vi "UiCharts24h_b2g2.vi"() -> ()   [LabVIEW 2011]
uses:
  Output - Cluster b2g2.ctl
  Input - Cluster b2g2.ctl
  <vilib>/Platform/TimedLoop/XDataNode/timing_clust.ctl
  <vilib>/Platform/TimedLoop/XDataNode/nitl_modes.ctl
  <vilib>/Platform/TimedLoop/XDataNode/wakeup.ctl
  <vilib>/addons/database/Connection.llb/DB Tools Open Connec (String).vi
  <vilib>/addons/database/Connection.llb/Conn Execute.vi
  <vilib>/addons/database/Recordset.llb/Rec Fetch Recordset Data (R).vi
  <vilib>/addons/database/Recordset.llb/Rec Destroy - Connection.vi
  <vilib>/Platform/TimedLoop/XDataNode/XDataNode.xnode
  <vilib>/addons/database/_DB Variant To Data/Database Variant To Data.xnode
  <vilib>/addons/database/NI_Database_API.lvlib
  <vilib>/Platform/TimedLoop/XDataNode/XDNodeRunTimeDep.lvlib
panel:
  in  "Output Var":refnum<k21>="ni.var.psp://10.27.40.21/variables - b2g2/data - network b2g2"
  in  "Input Var":refnum<k21>="ni.var.psp://10.27.40.21/variables - b2g2/input - network b2g2"
  in  "Tab Control":T1(tab)
  out "protocol":string[][](table)
  out "pH-Wert":dbl(graph)
  out "Temperaturregelung":T2(graph)
  out "Füllstandsregelung":T3(graph)
  out "Druckregelung":T4(graph)
  out "error out":errorcluster
  in  "stop":bool
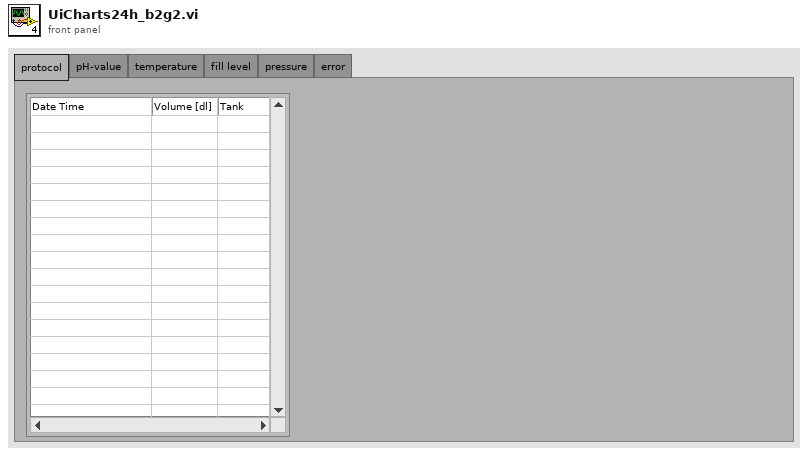
[diagram p1: front panel]
types:
  T1 = enum32{"protocol", "pH-value", "temperature", "fill level", "pressure", "error"}
  T2 = cluster{"Temp Soll [°C]":sgl, "TS-4 [°C]":dbl, dbl, dbl}
  T3 = cluster{"Füllstand Soll [l]":sgl, "FS-3 [l]":dbl, dbl}
  T4 = cluster{"Druck Soll [bar]":sgl, "DS-1 [bar]":dbl, dbl, dbl}
  T5 = typedef "Input - Cluster b2g2.ctl" = cluster{"V-13 [%]":u8, "V-15 [%]":u8, "Log-Target":bool, "P-4":bool, "P-4 Drehzahl [%]":u8, "Temperaturregelung":bool, "Überdruckregelung":bool, "Füllstandsregulierung":bool, "V-10":bool, "Log-Host":bool, "V-14":bool, "HS-1":bool, "Füllstand  P":sgl, "Füllstand I":sgl, "Füllstand D":sgl, "Füllstand Soll [l]":sgl, "Druck  P":sgl, "Druck I":sgl, "Druck D":sgl, "Druck Soll [bar]":sgl, "Temp Soll [°C]":sgl, "Dosierung":bool, "Dosiermenge [l]":sgl, "Dosiergeschw. [l/min]":sgl, "Tank":bool, "Hysterese [°C]":sgl, "MR Füllstandsüberwachung":bool, "Tank Füllstandsüberwachung":bool, "Log Target [ms]":u32, "Log Host [s]":u32, "Zirkulation EIN [min]":u8, "Zirkulation AUS [min]":u8, "Zirkulation":bool, "V-33":bool, "V-34":bool, "V-35":bool}
  T6 = typedef "Output - Cluster b2g2.ctl" = cluster{"DFS-1 [dl]":u64, "FS-3 [l]":dbl, "DFS-1 [l/min]":dbl, "DS-1 [bar]":dbl, "V-10 ZU":bool, "V-14 ZU":bool, "FS-1 [l]":dbl, "FS-2 [l]":dbl, "TS-4 [°C]":dbl, "HS-1":bool, "V-13 [%]":u8, "V-15 [%]":u8, "P-4 [%]":u8, "Dosierung":bool, "MR Max Füllstand":bool, "MR Min Füllstand":bool, "Dosiermenge [l]":sgl, "V-14 AUF":bool, "V-10 AUF":bool, "T-1 Max Füllstand":bool, "T-1 Min Füllstand":bool, "T-2 Max Füllstand":bool, "T-2 Min Füllstand":bool, "pHS-1 [pH]":dbl, "P-4 RUN":bool, "V-33 AUF":bool, "V-33 ZU":bool, "V-34 AUF":bool, "V-34 ZU":bool, "P-4 ERR":bool, "TS-5 [°C]":dbl, "V-35 AUF":bool, "V-35 ZU":bool}
  T7 = typedef "XDNodeRunTimeDep.lvlib/timing_clust.ctl" = cluster{"Expected End [f-1]":u64, "Actual End [f-1]":u64, "Finished Late? [f-1]":bool, "Expected End [i-1]":u64, "Actual End [i-1]":u64, "Finished Late? [i-1]":bool, "Expected Start [i]":u64, "Actual Start [i]":u64, "Expected Start [f]":u64, "Actual Start [f]":u64, "Source Name":string, "Structure Name":string, "Period":i64, "Deadline":i64, "Offset":i64, "Start":i64, "Priority":i32, "Timeout":i32, "Mode":T8, "Wakeup Reason":T9, "Error":errorcluster, "Source Type":string, "Secondary Source Type":string, "Global End Time":u64, "Global Start Time":u64, "Frame Duration":u64, "Iteration Duration":u64, "Assigned CPU":i32, "I/O Scan Engine Mode":u32}
  T8 = typedef "XDNodeRunTimeDep.lvlib/nitl_modes.ctl" = enum32{"No Change", "Process missed periods, maintain original phase", "Discard missed periods, maintain original phase", "Process missed periods, ignore original phase", "Discard missed periods, ignore original phase"}
  T9 = typedef "XDNodeRunTimeDep.lvlib/wakeup.ctl" = enum32{"Normal", "Aborted", "Asynchronous wakeup", "Timing source error", "Timed loop error", "Timeout"}
  T10 = typedef "NI_Database_API.lvlib/Conn ObjectReference.ctl" = refnum<k1>
  T11 = typedef "NI_Database_API.lvlib/Rec ObjectReference.ctl" = refnum<k1>
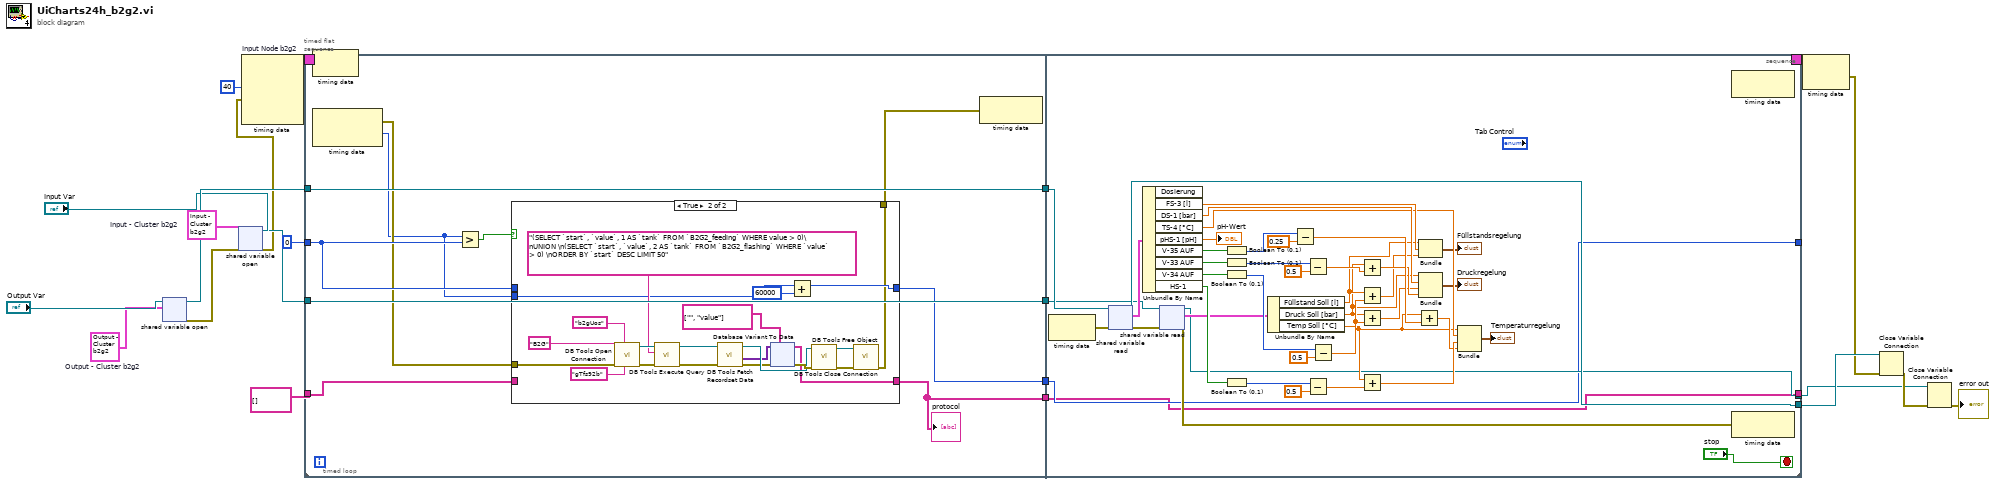
[diagram p0: block diagram]
diagram:
  w13 = T5 {"V-13 [%]"=0, "V-15 [%]"=0, "Log-Target"=FALSE, "P-4"=FALSE, "P-4 Drehzahl [%]"=0, "Temperaturregelung"=FALSE, "Überdruckregelung"=FALSE, "Füllstandsregulierung"=FALSE, "V-10"=FALSE, "Log-Host"=FALSE, "V-14"=FALSE, "HS-1"=FALSE, "Füllstand  P"=0.0, "Füllstand I"=0.0, "Füllstand D"=0.0, "Füllstand Soll [l]"=0.0, "Druck  P"=0.0, "Druck I"=0.0, "Druck D"=0.0, "Druck Soll [bar]"=0.0, "Temp Soll [°C]"=0.0, "Dosierung"=FALSE, "Dosiermenge [l]"=0.0, "Dosiergeschw. [l/min]"=0.0, "Tank"=FALSE, "Hysterese [°C]"=0.0, "MR Füllstandsüberwachung"=FALSE, "Tank Füllstandsüberwachung"=FALSE, "Log Target [ms]"=0, "Log Host [s]"=0, "Zirkulation EIN [min]"=0, "Zirkulation AUS [min]"=0, "Zirkulation"=FALSE, "V-33"=FALSE, "V-34"=FALSE, "V-35"=FALSE}  # Input - Cluster b2g2
  w17 = T6 {"DFS-1 [dl]"=0, "FS-3 [l]"=0.0, "DFS-1 [l/min]"=0.0, "DS-1 [bar]"=0.0, "V-10 ZU"=FALSE, "V-14 ZU"=FALSE, "FS-1 [l]"=0.0, "FS-2 [l]"=0.0, "TS-4 [°C]"=0.0, "HS-1"=FALSE, "V-13 [%]"=0, "V-15 [%]"=0, "P-4 [%]"=0, "Dosierung"=FALSE, "MR Max Füllstand"=FALSE, "MR Min Füllstand"=FALSE, "Dosiermenge [l]"=0.0, "V-14 AUF"=FALSE, "V-10 AUF"=FALSE, "T-1 Max Füllstand"=FALSE, "T-1 Min Füllstand"=FALSE, "T-2 Max Füllstand"=FALSE, "T-2 Min Füllstand"=FALSE, "pHS-1 [pH]"=0.0, "P-4 RUN"=FALSE, "V-33 AUF"=FALSE, "V-33 ZU"=FALSE, "V-34 AUF"=FALSE, "V-34 ZU"=FALSE, "P-4 ERR"=FALSE, "TS-5 [°C]"=0.0, "V-35 AUF"=FALSE, "V-35 ZU"=FALSE}  # Output - Cluster b2g2
  n1 = shared-variable-open("Output Var", w17) -> (w16:refnum<k21>, w10:errorcluster)  [unwired: 2 in]
  n2 = shared-variable-open("Input Var", w10, w13) -> (w11:refnum<k21>, w9:errorcluster)  [unwired: 1 in]
  n3 = node-c288 "Input Node b2g2"(40 ("Priority"), w9) -> (w2:T7)  [unwired: 2 in]
  n4 = timed-loop {
    timing: w2 -> [_]
    timing-out: [_] -> w1
    tunnel: w16 -> [w26]
    tunnel: [w25] -> w15
    tunnel: w11 -> [w24]
    tunnel: [w23] -> w7
    tunnel: i64 0 -> [w22]
    tunnel: [w21] -> _
    tunnel: string[][] [] ("data") -> [w20]
    tunnel: [w19] -> _
    stop <- "stop" stop-if-true
    n5 = timed-sequence {
      timing: _ -> [_]
      timing-out: _ -> [_]
      tunnel: w26 -> [w38]
      tunnel: [w37] -> w25
      tunnel: w24 -> [w36]
      tunnel: [w35] -> w23
      tunnel: w22 -> [w30]
      tunnel: [w29] -> w21
      tunnel: w20 -> [w28]
      tunnel: [w27] -> w19
      n6 = timed-flat-sequence {
        tunnel: w36 -> [w47]
        tunnel: w38 -> [w48]
        tunnel: [w48] -> w34
        tunnel: [w47] -> w33
        tunnel: [w45] -> w32
        tunnel: [w43] -> w31
        tunnel: w30 -> [w44]
        tunnel: w28 -> [w42]
        tunnel: [w164] -> w37
        tunnel: [w126] -> w35
        tunnel: w34 -> [w165]
        tunnel: w33 -> [w131]
        tunnel: w32 -> [w125]
        tunnel: w31 -> [w124]
        tunnel: [w125] -> w29
        tunnel: [w124] -> w27
        frame #0 {
          n7 = node-c288() -> (w41:errorcluster, w39:i64)  [unwired: 1 in]
          n8 = Greater?(x=w39, y=w44) -> (0:w46:bool)
          n9 = case shown="True" w46 {
            tunnel: [w50 w60] -> w43
            tunnel: [w51 w58] -> w45
            tunnel: w44 -> [w51 _]
            tunnel: w39 -> [_ w59]
            tunnel: w42 -> [w50 _]
            tunnel: w41 -> [w49 w56]
            tunnel: [w49 w55] -> w40
            frame False {
            }
            frame True {
              n10 = call-poly <vilib>:"DB Tools Open Connection.vi"("password"="gTfs92b", "userID"="b2gUos", "error in (no error)"=w56, "connection information"="B2G") -> ("error out"=w67:errorcluster, "connection reference"=w68:T10)  [unwired: 4 in]
              n11 = call-poly <vilib>:"DB Tools Execute Query.vi"("error in (no error)"=w67, "SQL query"="(SELECT `start`, `value`, 1 AS `tank` FROM `B2G2_feeding` WHERE value > 0)\nUNION \n(SELECT `start`, `value`, 2 AS `tank` FROM `B2G2_flashing` WHERE `value` > 0) \nORDER BY `start` DESC LIMIT 50", "connection reference"=w68) -> ("error out"=w64:errorcluster, "recordset reference"=w62:T11)  [unwired: 5 in]
              n12 = call-poly <vilib>:"DB Tools Fetch Recordset Data.vi"("error in (no error)"=w64, "recordset reference"=w62) -> ("error out"=w65:errorcluster, "recordset data"=w66:variant[][], "recordset reference out"=w69:T11)  [unwired: 3 in]
              n13 = xnode "Database Variant To Data"("database variant"=w66, "error in"=w65, "type"=string[][] [["", "value"]] ("columns")) -> ("data"=w60:string[][], "error out"=w71:errorcluster)
              n14 = Add(x=w59, y=i64 60000) -> (x+y=w58:i64)
              n15 = call-poly <vilib>:"DB Tools Free Object.vi"("error in (no error)"=w71, "recordset reference"=w69) -> ("error out"=w72:errorcluster, "connection reference"=w70:T10)  [unwired: 8 in]
              n16 = call <vilib>:"DB Tools Close Connection.vi"("error in (no error)"=w72, "connection reference"=w70) -> ("error out"=w55:errorcluster)  [unwired: 5 in]
            }
          }
          "protocol" <- w43
          n17 = node-c288(w40) -> ()  [unwired: 1 out]
        }
        frame #1 {
          n18 = node-c288() -> (w134:errorcluster)  [unwired: 1 in]
          n19 = shared-variable-read(w165, w134) -> (w164:refnum<k21>, w133:errorcluster, w163:T6)  [unwired: 1 out]
          n20 = Unbundle By Name(w163) -> ("FS-3 [l]"=w162:dbl, "DS-1 [bar]"=w161:dbl, "TS-4 [°C]"=w160:dbl, "pHS-1 [pH]"=→"pH-Wert":dbl, "V-35 AUF"=w156:bool, "V-33 AUF"=w158:bool, "V-34 AUF"=w157:bool, "HS-1"=w155:bool)  [unwired: 1 out]
          n21 = shared-variable-read(w131, w133) -> (w126:refnum<k21>, w132:errorcluster, w130:T5)  [unwired: 1 out]
          n22 = Boolean To (0,1)(Boolean=w156) -> (0, 1=w148:i16)
          n23 = Boolean To (0,1)(Boolean=w158) -> (0, 1=w139:i16)
          n24 = Boolean To (0,1)(Boolean=w157) -> (0, 1=w138:i16)
          n25 = Boolean To (0,1)(Boolean=w155) -> (0, 1=w151:i16)
          n26 = Unbundle By Name(w130) -> ("Füllstand Soll [l]"=w129:sgl, "Druck Soll [bar]"=w127:sgl, "Temp Soll [°C]"=w128:sgl)
          n27 = Subtract(x=w148, y=0.25) -> (x-y=w150:dbl)
          n28 = Subtract(x=w139, y=0.5) -> (x-y=w146:dbl)
          n29 = Subtract(x=w151, y=0.5) -> (x-y=w154:dbl)
          n30 = Subtract(x=w138, y=0.5) -> (x-y=w140:dbl)
          n31 = Add(x=w127, y=w146) -> (x+y=w144:dbl)
          n32 = Add(x=w129, y=w140) -> (x+y=w141:dbl)
          n33 = Add(x=w127, y=w140) -> (x+y=w142:dbl)
          n34 = Add(x=w128, y=w154) -> (x+y=w153:dbl)
          n35 = Add(x=w128, y=w150) -> (x+y=w147:dbl)
          n36 = Bundle("Füllstand Soll [l]"=w129, "FS-3 [l]"=w162, w141) -> (→"Füllstandsregelung":T3)  [unwired: 1 in]
          n37 = Bundle("Druck Soll [bar]"=w127, "DS-1 [bar]"=w161, w142, w144) -> (→"Druckregelung":T4)  [unwired: 1 in]
          n38 = Bundle("Temp Soll [°C]"=w128, "TS-4 [°C]"=w160, w153, w147) -> (→"Temperaturregelung":T2)  [unwired: 1 in]
          n39 = node-c288(w132) -> ()  [unwired: 1 out]
        }
      }
    }
    n40 = node-c288() -> ()  [unwired: 1 in, 1 out]
    n41 = node-c288() -> ()  [unwired: 1 in, 1 out]
  }
  n42 = node-c288(w1) -> (w14:errorcluster)
  n43 = Close Variable Connection(8:w14, 11:w15) -> (0:w8:errorcluster)
  n44 = Close Variable Connection(8:w8, 11:w7) -> (0:→"error out":errorcluster)
